vi "4Pi Focus Lock - Img Norm.vi"(8 "error in":errorcluster, 11 "Image In":T1) -> (0 "error out":errorcluster, 3 "Image Dst Out":T1)   [LabVIEW 2016]
uses:
  <vilib>/vision/Image Controls.llb/IMAQ Image.ctl
  <vilib>/vision/NI_Vision_Development_Module.lvlib
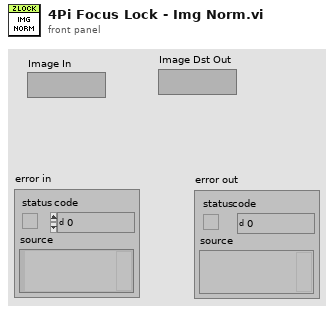
[diagram p1: front panel]
types:
  T1 = typedef "IMAQ Image.ctl" = refnum<image>
  T2 = cluster{"histogram":u32[], "Minimal Value":sgl, "Maximal Value":sgl, "Starting Value":sgl, "Interval Width":sgl, "Mean Value":sgl, "Standard  Variation":sgl, "Area (pixels)":i32}
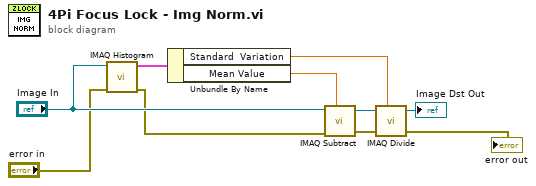
[diagram p0: block diagram]
diagram:
  n1 = call "IMAQ Histogram"("error in (no error)"="error in", "Image"="Image In") -> ("error out"=w5:errorcluster, "Histogram Report"=w10:T2)  [unwired: 8 in]
  n2 = Unbundle By Name(w10) -> ("Standard  Variation"=w8:sgl, "Mean Value"=w7:sgl)
  n3 = call "IMAQ Subtract"("Image Src A"="Image In", "Constant"=w7, "error in (no error)"=w5) -> ("Image Dst Out"=w9:T1, "error out"=w4:errorcluster)  [unwired: 4 in]
  n4 = call "IMAQ Divide"("Image Src A"=w9, "Constant"=w8, "error in (no error)"=w4) -> ("Image Dst Out"=→"Image Dst Out":T1, "error out"=→"error out":errorcluster)  [unwired: 4 in]
